vi "on_value_change.vi"(8 "error in (no error)":errorcluster, 9 "NewVal":i32, 10 "OldVal":i32, 11 "window in":refnum<class "rywindow.lvclass">) -> (0 "error out":errorcluster, 3 "window out":refnum<class "rywindow.lvclass">)   [LabVIEW 2017, in "rywindow.lvclass"]
uses:
  rywindow.lvclass
  rywindow.lvclass/rywindow.ctl
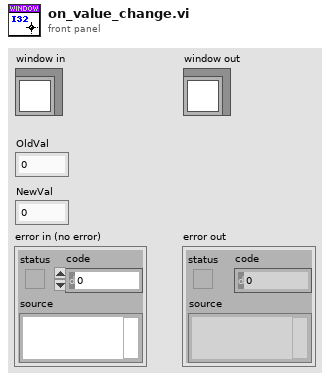
[diagram p1: front panel]
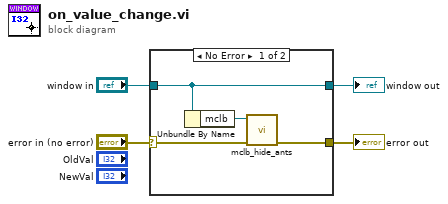
[diagram p0: block diagram]
diagram:
  n1 = case shown="No Error" "error in (no error)" {
    selector: "error in (no error)" -> [w8 w10]
    tunnel: [w6 w10] -> w3
    tunnel: [w7 w9] -> w1
    tunnel: "window in" -> [w7 w9]
    frame No Error {
      n2 = Unbundle By Name(w7) -> ("mclb"=w5:refnum<vi>)
      n3 = call "mclb_hide_ants.vi"("error in (no error)"=w8, "mclb in"=w5) -> ("error out"=w6:errorcluster)  [unwired: 8 in, 1 out]
    }
    frame Error {
    }
  }
  "error out" <- w3
  "window out" <- w1
